vi "Create Dev Panel.vi"(11 "Dev Actor in":refnum<class "Dev Actor.lvclass">) -> (0 "error out":errorcluster, 3 "Dev Actor out":refnum<class "Dev Actor.lvclass">)   [LabVIEW 2021, in "Dev Actor.lvlib" / "Dev Actor.lvclass"]
uses:
  Dev Actor.lvclass
  Dev Panel/Dev Panel.lvclass
  C:/git/Dev-Actor/src/Helper Loop/Helper Loop/Helper Loop.lvclass
  Dev Actor.lvclass/Dev Actor.ctl
  Helper Loop/Helper Loop/Helper Loop.lvclass
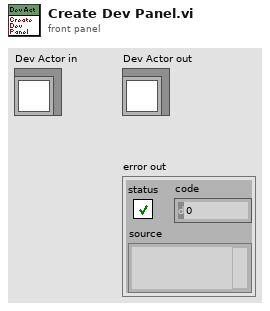
[diagram p1: front panel]
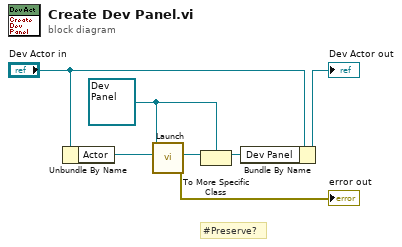
[diagram p0: block diagram]
diagram:
  w3 = refnum<class "Dev Panel.lvclass"> refnum ("Dev Panel.lvclass")
  # "#Preserve?"
  n1 = Unbundle By Name("Dev Actor in") -> ("Actor"=w5:refnum<class "Actor.lvclass">)
  n2 = call "Launch.vi"("Actor"=w5, "Helper Loop in"=w3) -> ("error out"=→"error out":errorcluster, "Helper Loop"=w1:refnum<class "Helper Loop.lvclass">)  [unwired: 8 in]
  n3 = To More Specific Class(target class=w3, reference=w1) -> (specific class reference=w4:refnum<class "Dev Panel.lvclass">)  [unwired: 1 in, 1 out]
  n4 = Bundle By Name(cluster="Dev Actor in", "Dev Panel"=w4) -> (→"Dev Actor out":refnum<class "Dev Actor.lvclass">)
